vi "Intake Logic.vi"() -> ()   [LabVIEW 2020]
uses:
  <vilib>/Rock Robotics/WPI/ThirdParty/Phoenix-LabVIEW/Motor Controller/Controls/CTRE_Phoenix_MotorControl_ControlMode.ctl
  <vilib>/Rock Robotics/WPI/ThirdParty/REV Robotics/REVLib/Typedef/Spark MAX Control Type.ctl
  <vilib>/Rock Robotics/WPI/Utilities/WPI_GetSetVariantRefNum.vi
  Robot Global Data.vi
  2017 Swerve Code/Swerve Global Variables.vi
  <vilib>/addons/control/pid/pid.llb/PID (DBL).vi
  <vilib>/addons/control/pid/NI_PID_pid.lvlib
  <vilib>/ptbypt/NI_PtbyPt.lvlib
panel:
  in  "Shooter Speed Threshold":dbl=50.0
  in  "Angle PID 2":T1={"proportional gain (Kc)"=0.03, "integral time (Ti, min)"=0.0, "derivative time (Td, min)"=0.0} {"derivative time (Td, min)" format="%.6f"; "integral time (Ti, min)" format="%.3f"; "proportional gain (Kc)" format="%.3f"}
  in  "output range 2":cluster{"output high":dbl, "output low":dbl}={"output high"=0.5, "output low"=-0.5} {"output low" format="%.2f"; "output high" format="%.2f"}
  in  "Shooter PID":T2={"P Gain"=0.0, "I Gain"=0.0, "D Gain"=0.0, "F Gain"=0.0, "I Zone"=0.0, "Min Output"=-1.0, "Max Output"=1.0}
  in  "Set PID":bool
  in  "ball sense voltage":dbl=3.8 format="%#_13g"
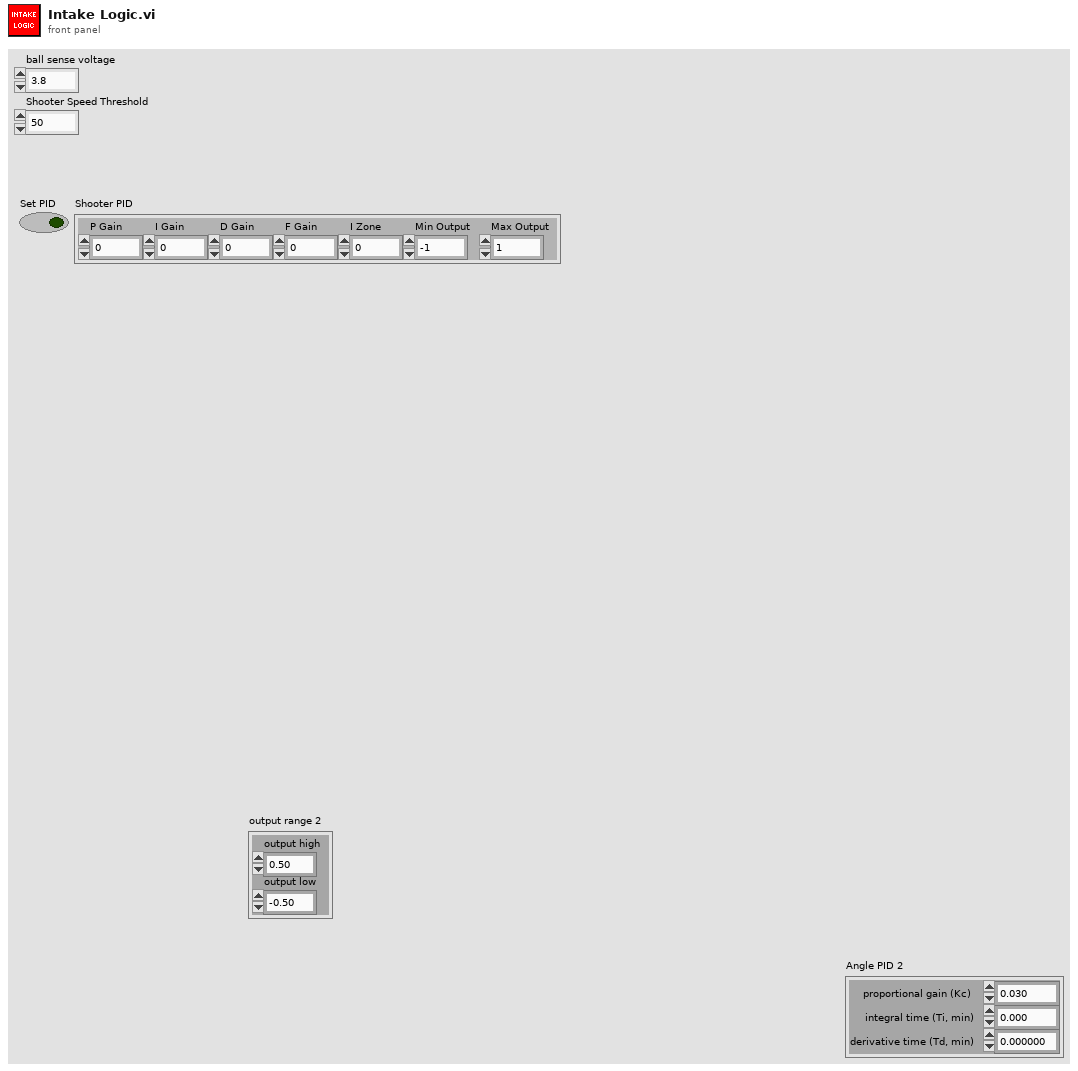
[diagram p1: front panel]
types:
  T1 = cluster{"proportional gain (Kc)":dbl, "integral time (Ti, min)":dbl, "derivative time (Td, min)":dbl}
  T2 = cluster{"P Gain":dbl, "I Gain":dbl, "D Gain":dbl, "F Gain":dbl, "I Zone":dbl, "Min Output":dbl, "Max Output":dbl}
  T3 = typedef "WPI_MotorControlDeviceRef.ctl" = cluster{"DeviceStatus":errorcluster, "Type":T4, "PWM":cluster{"PWM Channel":T5, "DeadBand":T6}, "CAN":cluster{"Device Number":u8, "SetOutput VI Ref":variant, "GetOutput VI Ref":variant, "Enable VI Ref":variant, "Disable VI Ref":variant, "Data":variant}, "Invert":bool, "DIO PWM":cluster{"PWM \"Enable\" Channel":T5, "DIOChannel":T7, "PWM Rate":dbl}}
  T4 = typedef "WPI_MotorControlType.ctl" = enum16{"PWM", "CAN", "DIO PWM"}
  T5 = typedef "FPGA_DIOPWMChannel.ctl" = enum8{"PWM 0", "PWM 1", "PWM 2", "PWM 3", "PWM 4", "PWM 5", "PWM 6", "PWM 7", "PWM 8", "PWM 9", "PWM MXP 0", "PWM MXP 1", "PWM MXP 2", "PWM MXP 3", "PWM MXP 4", "PWM MXP 5", "PWM MXP 6", "PWM MXP 7", "PWM MXP 8", "PWM MXP 9", "Invalid"}
  T6 = typedef "WPI_PWMDeadband.ctl" = cluster{"Name":string, "maxPositivePwm":i32, "minPositivePwm":i32, "centerPwm":i32, "maxNegativePwm":i32, "minNegativePwm":i32, "angularRange":u16}
  T7 = typedef "FPGA_DIOChannel.ctl" = enum8{"DIO 0", "DIO 1", "DIO 2", "DIO 3", "DIO 4", "DIO 5", "DIO 6", "DIO 7", "DIO 8", "DIO 9", "DIO MXP 0", "DIO MXP 1", "DIO MXP 2", "DIO MXP 3", "DIO MXP 4", "DIO MXP 5", "DIO MXP 6", "DIO MXP 7", "DIO MXP 8", "DIO MXP 9", "DIO MXP 10", "DIO MXP 11", "DIO MXP 12", "DIO MXP 13", "DIO MXP 14", "DIO MXP 15", "SPI Port CS1", "SPI Port CS2", "SPI Port CS3", "SPI Port MISO", "SPI Port MOSI", "Invalid"}
  T8 = typedef "WPI_AnalogChannelDevRef.ctl" = cluster{"DevStatus":errorcluster, "Analog Channel":T9}
  T9 = typedef "FPGA_AIChannel.ctl" = enum8{"AI 0", "AI 1", "AI 2", "AI 3", "AI MXP 0", "AI MXP 1", "AI MXP 2", "AI MXP 3", "Invalid"}
  T10 = typedef "Spark MAX Control Type.ctl" = enum16{"Percent VBus", "Voltage", "Velocity", "Position", "Smart Motion", "Current", "Smart Velocity"}
  T11 = typedef "CTRE_Phoenix_MotorControl_ControlMode.ctl" = u16
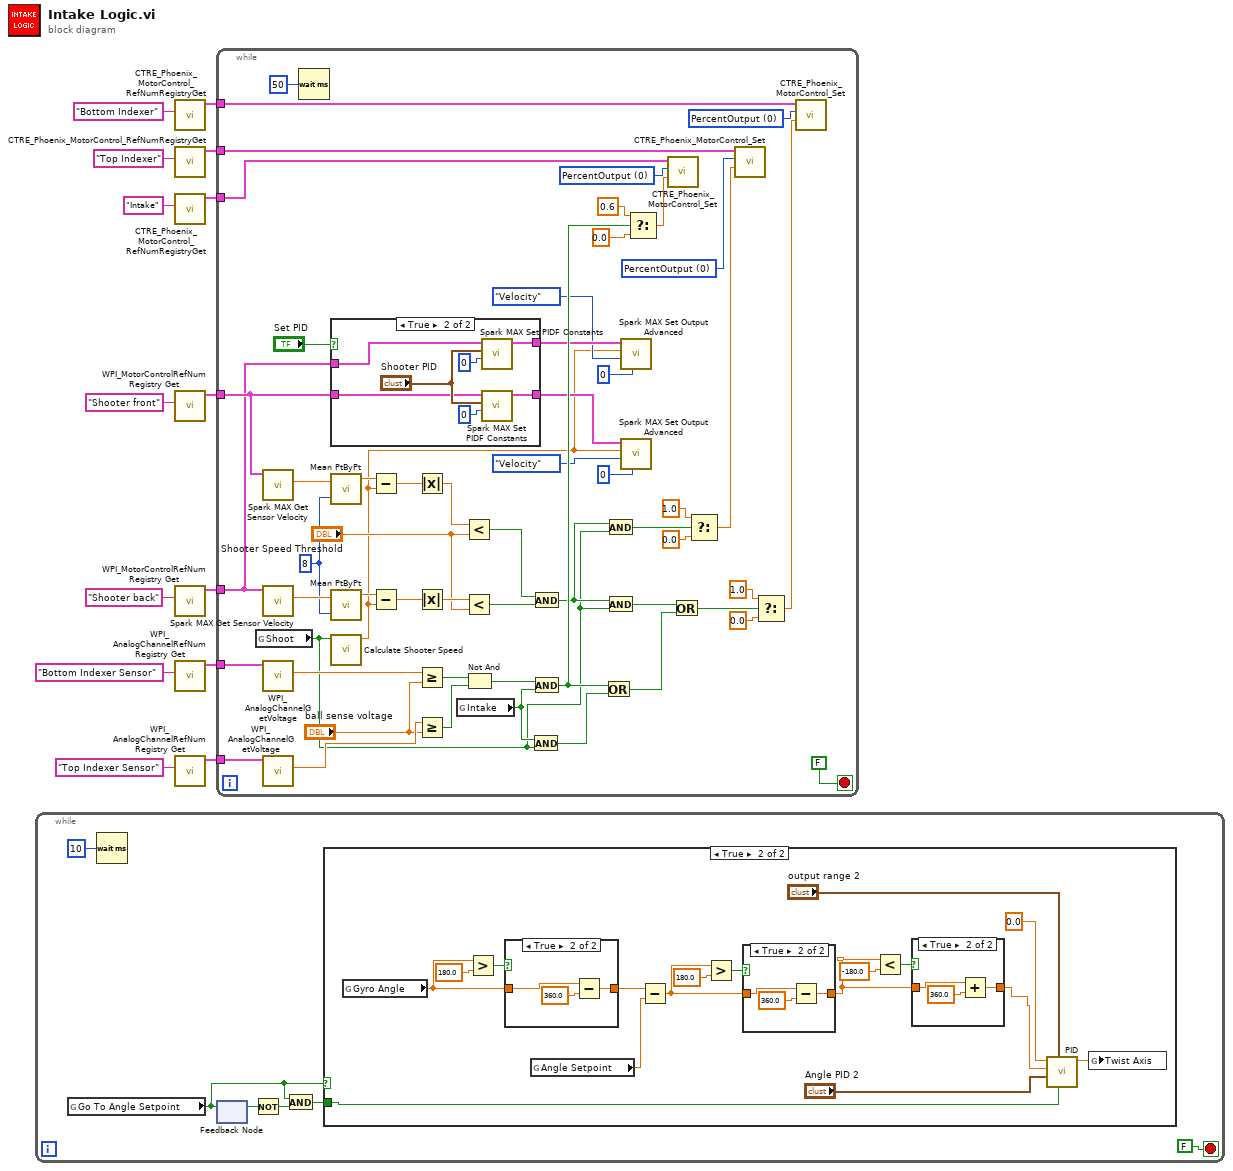
[diagram p0: block diagram]
diagram:
  n1 = while {
    stop <- FALSE stop-if-true
    n2 = global read "Robot Global Data.vi" "Go To Angle Setpoint"() -> (w16:bool)
    n3 = Wait (ms)(milliseconds to wait=u32 10) -> ()  [unwired: 1 out]
    n4 = feedback-in #1(w16) -> ()
    n5 = feedback #1() -> (w18:bool)  [unwired: 1 in]
    n6 = Not(x=w18) -> (.not. x?=w17:bool)
    n7 = And(x=w16, y=w17) -> (x .and. y?=w15:bool)
    n8 = case shown="True" w16 {
      tunnel: w15 -> [_ w28]
      frame False {
      }
      frame True {
        n9 = global read "Swerve Global Variables.vi" "Gyro Angle"() -> (w32:dbl)
        n10 = Greater?(x=w32, y=180.0) -> (0:w35:bool)
        n11 = case shown="True" w35 {
          tunnel: w32 -> [w46 w48]
          tunnel: [w46 w47] -> w34
          frame False {
          }
          frame True {
            n12 = Subtract(x=w48, y=360.0) -> (x-y=w47:dbl)
          }
        }
        n13 = global read "Robot Global Data.vi" "Angle Setpoint"() -> (w29:dbl)
        n14 = Subtract(x=w34, y=w29) -> (x-y=w25:dbl)
        n15 = Greater?(x=w25, y=180.0) -> (0:w26:bool)
        n16 = case shown="True" w26 {
          tunnel: w25 -> [w42 w44]
          tunnel: [w42 w43] -> w21
          frame False {
          }
          frame True {
            n17 = Subtract(x=w44, y=360.0) -> (x-y=w43:dbl)
          }
        }
        n18 = Less?(x=w21, y=-180.0) -> (x < y?=w23:bool)
        n19 = case shown="True" w23 {
          tunnel: w21 -> [w38 w40]
          tunnel: [w38 w39] -> w22
          frame False {
          }
          frame True {
            n20 = Add(x=w40, y=360.0) -> (x+y=w39:dbl)
          }
        }
        n21 = call-poly <vilib>:"PID.vi"("reinitialize? (F)"=w28, "output range"="output range 2", "PID gains"="Angle PID 2", "process variable"=w22, "setpoint"=0.0) -> ("output"=w30:dbl)  [unwired: 5 in, 1 out]
        n22 = global write "Swerve Global Variables.vi" "Twist Axis"(w30) -> ()
      }
    }
  }
  n23 = call <vilib>:"CTRE_Phoenix_MotorControl_RefNumRegistryGet.vi"("refnum name"="Bottom Indexer") -> ("PhoenixMotorControlDevRef"=w14:T3)  [unwired: 9 in, 1 out]
  n24 = call <vilib>:"CTRE_Phoenix_MotorControl_RefNumRegistryGet.vi"("refnum name"="Top Indexer") -> ("PhoenixMotorControlDevRef"=w9:T3)  [unwired: 9 in, 1 out]
  n25 = call <vilib>:"CTRE_Phoenix_MotorControl_RefNumRegistryGet.vi"("refnum name"="Intake") -> ("PhoenixMotorControlDevRef"=w11:T3)  [unwired: 9 in, 1 out]
  n26 = call <vilib>:"WPI_MotorControlRefNum Registry Get.vi"("refnum name"="Shooter front") -> ("MotorControlDevRef"=w1:T3)  [unwired: 9 in, 1 out]
  n27 = call <vilib>:"WPI_MotorControlRefNum Registry Get.vi"("refnum name"="Shooter back") -> ("MotorControlDevRef"=w2:T3)  [unwired: 9 in, 1 out]
  n28 = call <vilib>:"WPI_AnalogChannelRefNum Registry Get.vi"("refnum name"="Bottom Indexer Sensor") -> ("AIDeviceRef"=w5:T8)  [unwired: 9 in, 1 out]
  n29 = call <vilib>:"WPI_AnalogChannelRefNum Registry Get.vi"("refnum name"="Top Indexer Sensor") -> ("AIDeviceRef"=w6:T8)  [unwired: 9 in, 1 out]
  n30 = while {
    tunnel: w11 -> [w102]
    tunnel: w14 -> [w103]
    tunnel: w9 -> [w82]
    tunnel: w6 -> [w99]
    tunnel: w5 -> [w98]
    tunnel: w2 -> [w66]
    tunnel: w1 -> [w69]
    stop <- FALSE stop-if-true
    w54 = 8 ("sample length")
    w81 = T11 0 items=["PercentOutput"=0, "Position"=1, "Velocity"=2, "Current"=3, "Follower"=5, "MotionProfile"=6, "MotionMagic"=7, "MotionProfileArc"=10, "Disabled"=15] ("Control Mode")
    w100 = T11 0 items=["PercentOutput"=0, "Position"=1, "Velocity"=2, "Current"=3, "Follower"=5, "MotionProfile"=6, "MotionMagic"=7, "MotionProfileArc"=10, "Disabled"=15] ("Control Mode")
    w101 = T11 0 items=["PercentOutput"=0, "Position"=1, "Velocity"=2, "Current"=3, "Follower"=5, "MotionProfile"=6, "MotionMagic"=7, "MotionProfileArc"=10, "Disabled"=15] ("Control Mode")
    n31 = global read "Robot Global Data.vi" "Shoot"() -> (w50:bool)
    n32 = call <vilib>:"Spark MAX Get Sensor Velocity.vi"("MotorControlDevRef in"=w69) -> ("Sensor Velocity"=w58:dbl)  [unwired: 7 in, 3 out]
    n33 = call <vilib>:"Spark MAX Get Sensor Velocity.vi"("MotorControlDevRef in"=w66) -> ("Sensor Velocity"=w56:dbl)  [unwired: 7 in, 3 out]
    n34 = call <vilib>:"WPI_AnalogChannelGetVoltage.vi"("AIDeviceRef"=w98) -> ("Voltage"=w97:dbl)  [unwired: 8 in, 2 out]
    n35 = call <vilib>:"WPI_AnalogChannelGetVoltage.vi"("AIDeviceRef"=w99) -> ("Voltage"=w96:dbl)  [unwired: 8 in, 2 out]
    n36 = Wait (ms)(milliseconds to wait=u32 50) -> ()  [unwired: 1 out]
    n37 = case shown="True" "Set PID" {
      tunnel: w66 -> [w107 w113]
      tunnel: w69 -> [w106 w112]
      tunnel: [w106 w109] -> w75
      tunnel: [w107 w108] -> w76
      frame False {
      }
      frame True {
        n38 = call <vilib>:"Spark MAX Set PIDF Constants.vi"("PIDF Slot"=0, "PID Constants"="Shooter PID", "MotorControlDeviceRef"=w113) -> ("MotorControlDeviceRef"=w108:T3)  [unwired: 7 in, 1 out]
        n39 = call <vilib>:"Spark MAX Set PIDF Constants.vi"("PIDF Slot"=0, "PID Constants"="Shooter PID", "MotorControlDeviceRef"=w112) -> ("MotorControlDeviceRef"=w109:T3)  [unwired: 7 in, 1 out]
      }
    }
    n40 = call <vilib>:"Mean PtByPt.vi"("x"=w58, "sample length"=w54) -> ("mean"=w57:dbl)  [unwired: 2 in, 1 out]
    n41 = call <vilib>:"Mean PtByPt.vi"("x"=w56, "sample length"=w54) -> ("mean"=w55:dbl)  [unwired: 2 in, 1 out]
    n42 = call "Calculate Shooter Speed.vi"("Shoot"=w50) -> ("Shooter Speed out"=w51:dbl)  [unwired: 10 in]
    n43 = Subtract(x=w57, y=w51) -> (x-y=w68:dbl)
    n44 = Subtract(x=w55, y=w51) -> (x-y=w65:dbl)
    n45 = Absolute Value(x=w68) -> (abs(x)=w67:dbl)
    n46 = Absolute Value(x=w65) -> (abs(x)=w64:dbl)
    n47 = Greater Or Equal?(x=w97, y="ball sense voltage") -> (x >= y?=w93:bool)
    n48 = Greater Or Equal?(x=w96, y="ball sense voltage") -> (x >= y?=w94:bool)
    n49 = global read "Robot Global Data.vi" "Intake"() -> (w79:bool)
    n50 = Less?(x=w67, y="Shooter Speed Threshold") -> (x < y?=w62:bool)
    n51 = Less?(x=w64, y="Shooter Speed Threshold") -> (x < y?=w61:bool)
    n52 = Not And(1:w94, 2:w93) -> (0:w78:bool)
    n53 = And(x=w79, y=w50) -> (x .and. y?=w86:bool)
    n54 = And(x=w62, y=w61) -> (x .and. y?=w52:bool)
    n55 = And(x=w78, y=w79) -> (x .and. y?=w80:bool)
    n56 = Or(x=w80, y=w86) -> (x .or. y?=w60:bool)
    n57 = And(x=w52, y=w50) -> (x .and. y?=w70:bool)
    n58 = And(x=w52, y=w50) -> (x .and. y?=w53:bool)
    n59 = call <vilib>:"Spark MAX Set Output Advanced.vi"("PIDF Slot (0)"=0, "Control Mode"=Spark_MAX_Control_Type."Velocity", "Setpoint"=w51, "MotorControlDevRef"=w76) -> ()  [unwired: 6 in, 2 out]
    n60 = call <vilib>:"Spark MAX Set Output Advanced.vi"("PIDF Slot (0)"=0, "Control Mode"=Spark_MAX_Control_Type."Velocity", "Setpoint"=w51, "MotorControlDevRef"=w75) -> ()  [unwired: 6 in, 2 out]
    n61 = Select(t=0.6, s=w80, f=0.0) -> (s? t:f=w85:dbl)
    n62 = call <vilib>:"CTRE_Phoenix_MotorControl_Set.vi"("Output"=w85, "Control Mode"=w101, "PhoenixMotorControlDevRef"=w102) -> ()  [unwired: 7 in, 2 out]
    n63 = Or(x=w53, y=w60) -> (x .or. y?=w59:bool)
    n64 = Select(t=1.0, s=w70, f=0.0) -> (s? t:f=w83:dbl)
    n65 = call <vilib>:"CTRE_Phoenix_MotorControl_Set.vi"("Output"=w83, "Control Mode"=w81, "PhoenixMotorControlDevRef"=w82) -> ()  [unwired: 7 in, 2 out]
    n66 = Select(t=1.0, s=w59, f=0.0) -> (s? t:f=w84:dbl)
    n67 = call <vilib>:"CTRE_Phoenix_MotorControl_Set.vi"("Output"=w84, "Control Mode"=w100, "PhoenixMotorControlDevRef"=w103) -> ()  [unwired: 7 in, 2 out]
  }
